vi "Diagnostic Init.vi"(8 "error in (no error)":errorcluster, 11 "CAP-USB-1 in":refnum<class "CAP-USB-1.lvclass">) -> (0 "error out":errorcluster, 3 "CAP-USB-1 out":refnum<class "CAP-USB-1.lvclass">)   [LabVIEW 2014]
uses:
  API/CAP-USB/CAP-USB.lvlib
  CAP-USB-1.lvclass
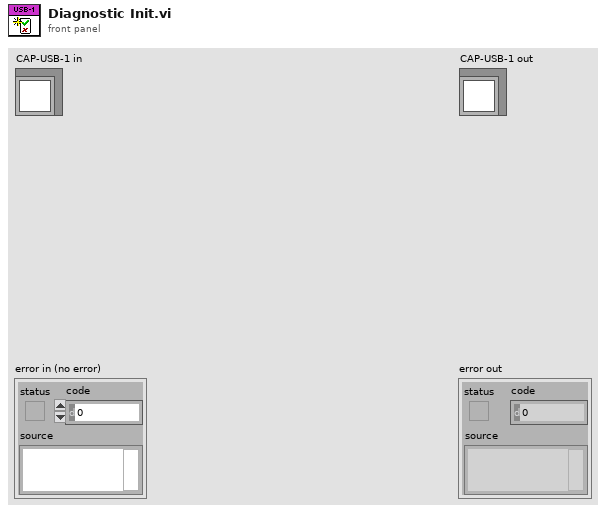
[diagram p1: front panel]
types:
  T1 = cluster{"Entradas":bool[], "Salidas":bool[], "Valor Encoder":u16, "Valor Transductores":u16[], "Orden Transd":u32[]}[]
  T2 = cluster{"Entradas":bool[], "Salidas":bool[], "Valor Encoder":u16, "Valor Transductores":u16[], "Orden Transd":u32[]}
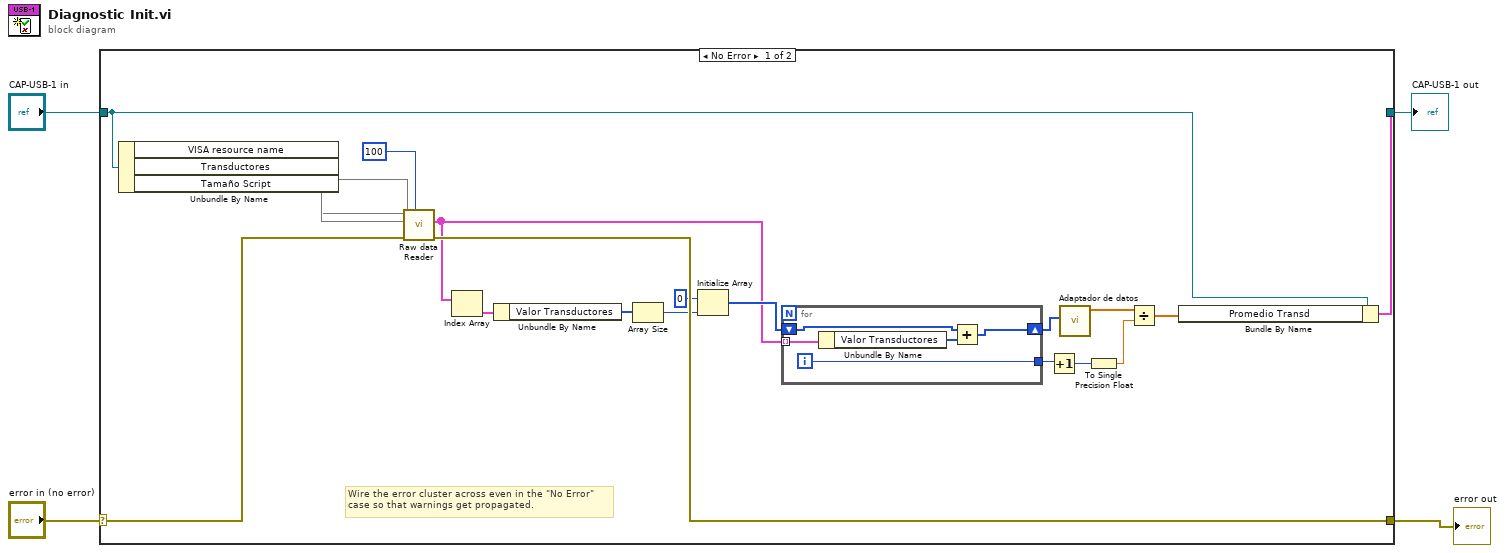
[diagram p0: block diagram]
diagram:
  n1 = case shown="No Error" "error in (no error)" {
    selector: "error in (no error)" -> [w22 w31]
    tunnel: [w21 w31] -> w3
    tunnel: [w9 w30] -> w1
    tunnel: "CAP-USB-1 in" -> [w10 w30]
    frame No Error {
      # "Wire the error cluster across even in the \"No Error\"\ncase so that warnings get propagated."
      n2 = Unbundle By Name(w10) -> ("VISA resource name"=w6, "Transductores"=w24, "Tamaño Script"=w23)
      n3 = call "Raw data Reader.vi"("Num de tramas"=100, "error in (no error)"=w22, "Tamaño Script"=w23, "TRANSDUCTORES"=w24, "VISA Refnum in"=w6) -> ("error out"=w21:errorcluster, "Raw data"=w17:T1)  [unwired: 2 in, 1 out]
      n4 = Index Array(array=w17) -> (element=w16:T2)  [unwired: 1 in]
      n5 = Unbundle By Name(w16) -> ("Valor Transductores"=w15:u16[])
      n6 = Array Size(array=w15) -> (size(s)=w14:i32)
      n7 = Initialize Array(u16 0, w14) -> (w18:u16[])
      n8 = for {
        tunnel: w17 -> [w29] mode=indexing
        shift-right: [w26] -> w8
        shift-left: w18 -> [w28]
        tunnel: [w25] -> w13
        i -> [w25]
        n9 = Unbundle By Name(w29) -> ("Valor Transductores"=w27:u16[])
        n10 = Add(x=w28, y=w27) -> (x+y=w26:u16[])
      }
      n11 = Increment(x=w13) -> (x+1=w12:i32)
      n12 = call "Adaptador de datos.vi"("Transductores"=w8) -> ("Transductores"=w7:sgl[])  [unwired: 8 in, 2 out]
      n13 = To Single Precision Float(number=w12) -> (single precision float=w11:sgl)
      n14 = Divide(x=w7, y=w11) -> (x/y=w5:sgl[])
      n15 = Bundle By Name(cluster=w10, "Promedio Transd"=w5) -> (w9:cluster{})
    }
    frame Error {
    }
  }
  "error out" <- w3
  "CAP-USB-1 out" <- w1
